vi "Check Close.vi"(11 "DaqControl in":T1) -> (1 "Stop":bool, 3 "DaqControl out":T1)   [LabVIEW 2020, in "VolatusDaq.lvlib" / "DaqControl.lvclass"]
uses:
  DaqControl.lvclass
  DaqControl.lvclass/DaqControl.ctl
  Value Update.ctl
  Sequence Action.ctl
  VolatusDaq.lvlib
  Loop Data.ctl
  Seq Cmd Type.ctl
  Seq Action Type.ctl
  Seq Cmd.ctl
  Signal Type.ctl
  Volatus/Event API/EventAPI.lvclass
  VolatusData/DataHandlerAPI/DataHandlerAPI.lvclass
  Sequence.ctl
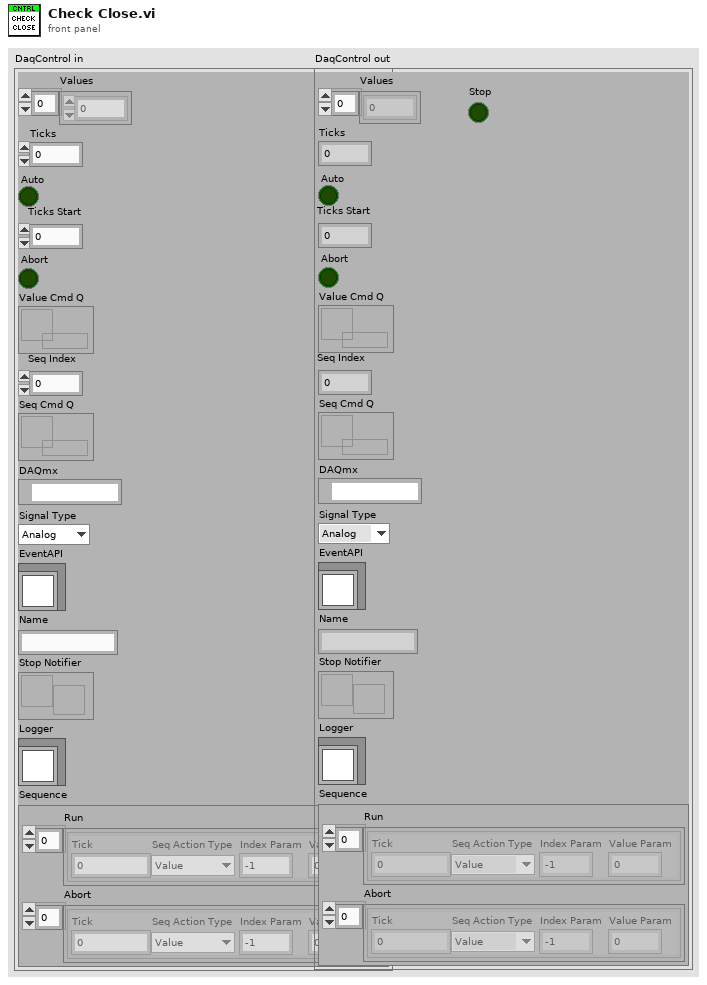
[diagram p1: front panel]
types:
  T1 = typedef "VolatusDaq.lvlib/DaqControl.lvclass/Loop Data.ctl" = cluster{"Values":dbl[], "Ticks":u32, "Auto":bool, "Ticks Start":u32, "Abort":bool, "Value Cmd Q":refnum<queue>, "Seq Index":i32, "Seq Cmd Q":refnum<queue>, "DAQmx":refnum<k21>, "Signal Type":T2, "EventAPI":refnum<class "EventAPI.lvclass">, "Name":string, "Stop Notifier":refnum<notifier>, "Logger":refnum<class "DataHandlerAPI.lvclass">, "Sequence":T3}
  T2 = typedef "VolatusDaq.lvlib/Signal Type.ctl" = enum16{"Analog", "Digital"}
  T3 = typedef "VolatusDaq.lvlib/Sequence.ctl" = cluster{"Run":T4[], "Abort":T4[]}
  T4 = typedef "VolatusDaq.lvlib/Sequence Action.ctl" = cluster{"Tick":u32, "Seq Action Type":T5, "Index Param":i32, "Value Param":dbl}
  T5 = typedef "VolatusDaq.lvlib/Seq Action Type.ctl" = enum16{"Value", "Stop"}
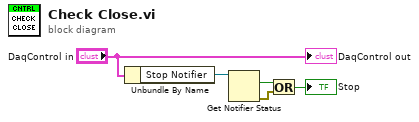
[diagram p0: block diagram]
diagram:
  n1 = Unbundle By Name("DaqControl in") -> ("Stop Notifier"=w4:refnum<notifier>)
  n2 = Get Notifier Status(notifier=w4) -> (current notification=w3:bool, error out=w1:errorcluster)  [unwired: 1 in, 3 out]
  n3 = Or(x=w3, y=w1) -> (x .or. y?=→"Stop":bool)
  "DaqControl out" <- "DaqControl in"
